vi "Master Ready For Data.vi"() -> ()   [LabVIEW 2016]
panel:
  out "Master Ready":bool
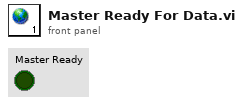
[diagram p1: front panel]
diagram:
